vi "GetRawDataFilePaths.vi"(11 "Results file or Folder":path) -> (3 "RawDataFilePaths":string[](array[string]), 5 "RowNumbers":i32[](array[numeric]))   [LabVIEW 2015]
uses:
  Globals/Constants_global.vi
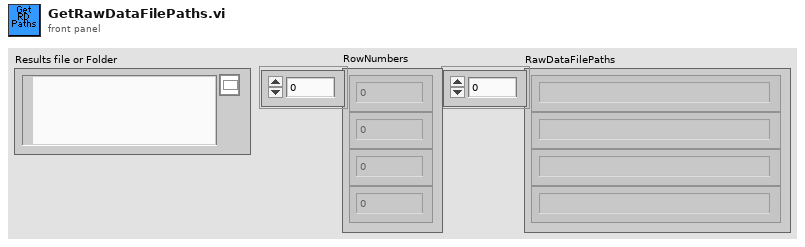
[diagram p1: front panel]
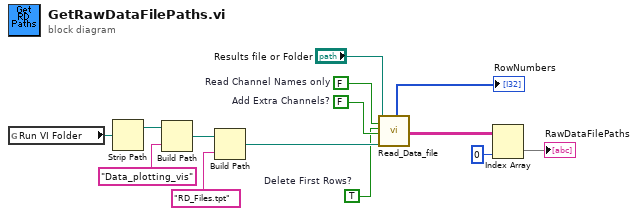
[diagram p0: block diagram]
diagram:
  w1 = TRUE  # Delete First Rows?
  w10 = FALSE  # Add Extra Channels?
  w9 = FALSE  # Read Channel Names only
  n1 = global read "Constants_global.vi" "Run VI Folder"() -> (w6:path)
  n2 = Strip Path(path=w6) -> (stripped path=w5:path)  [unwired: 1 out]
  n3 = Build Path(base path=w5, name or relative path="Data_plotting_vis") -> (appended path=w4:path)
  n4 = Build Path(base path=w4, name or relative path="RD_Files.tpt") -> (appended path=w8:path)
  n5 = call "Read_Data_file.vi"("Results file"="Results file or Folder", "Read Channel Names only"=w9, "Delete First Rows?"=w1, "Add Extra Channels?"=w10, "Template File"=w8) -> ("Row numbers"=→"RowNumbers":i32[], "Channel Values Out"=w14:string[][])  [unwired: 1 in, 12 out]
  n6 = Index Array(array=w14, index (col)=0 ("index (row)")) -> (element=→"RawDataFilePaths":string[])  [unwired: 1 in]
